vi "Idle_Password.vi"(2 "Called?":bool=TRUE) -> (0 "Correct?":bool, 1 "Access Level":i32)   [LabVIEW 2012]
uses:
  WVDIAL_GlobalVariables.vi
  <vilib>/Utility/miscctls.llb/LVPointTypeDef.ctl
  <vilib>/Utility/miscctls.llb/LVRectTypeDef.ctl
panel:
  in  "Cancel":bool
  in  "Password":string
  in  "Set Password":bool
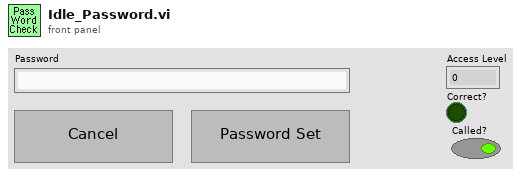
[diagram p1: front panel]
types:
  T1 = typedef "LVPointTypeDef.ctl" = cluster{"Horizontal":i16, "Vertical":i16}
  T2 = typedef "LVRectTypeDef.ctl" = cluster{"Left":i16, "Top":i16, "Right":i16, "Bottom":i16}
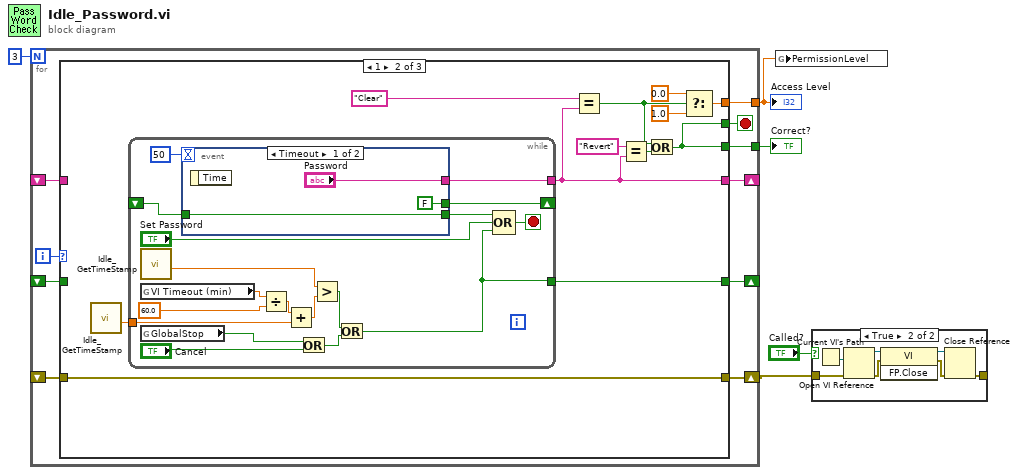
[diagram p0: block diagram]
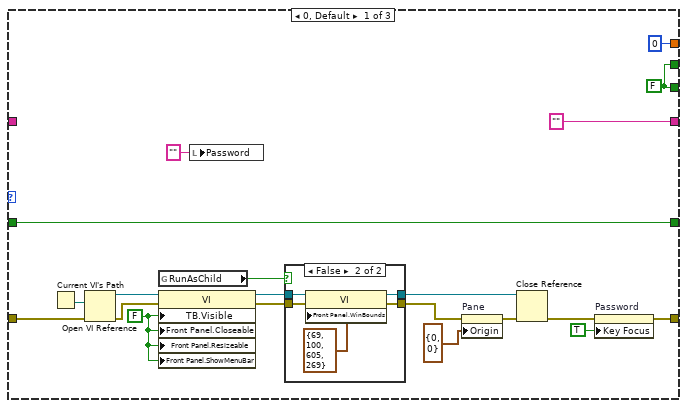
[diagram p3: hidden frame]
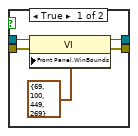
[diagram p4: hidden frame]
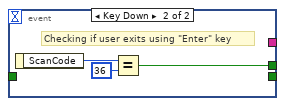
[diagram p5: hidden frame]
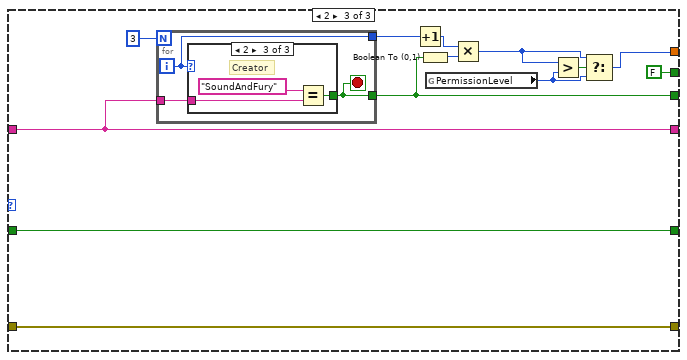
[diagram p6: hidden frame]
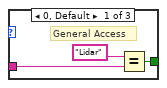
[diagram p7: hidden frame]
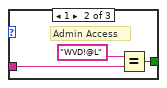
[diagram p8: hidden frame]
diagram:
  n1 = for {
    N: 3 -> [_]
    shift-right: [w14] -> _
    shift-left: _ -> [w11]
    shift-right: [w13] -> _
    shift-left: _ -> [w12]
    shift-right: [w9] -> w2
    shift-left: _ -> [w10]
    tunnel: [w8] -> w3
    tunnel: [w7] -> w4
    i -> [w15]
    stop <- w6 stop-if-true
    n2 = case shown="1" w15 {
      tunnel: ["" ("Comment") w53 w93] -> w14
      tunnel: [w32 w56 w94] -> w13
      tunnel: w12 -> [w32 _ w94]
      tunnel: w11 -> [_ _ w93]
      tunnel: w10 -> [w31 w46 w82]
      tunnel: [w17 w46 w82] -> w9
      tunnel: [w28 w47 w89] -> w7
      tunnel: [0 w51 w85] -> w8
      tunnel: [w28 w47 FALSE] -> w6
      frame 0, Default {
        w28 = FALSE
        w35 = FALSE ("Tool Bar:Visible")
        n3 = Current VI's Path() -> (path=w34:path)
        n4 = Open VI Reference(vi path=w34, error in (no error)=w31) -> (vi reference=w20:refnum<vi>, error out=w19:errorcluster)  [unwired: 4 in]
        n5 = global read "WVDIAL_GlobalVariables.vi" "RunAsChild"() -> (w21:bool)
        n6 = property class="VI"(reference=w20, error in=w19, "TB.Visible"=w35, "Front Panel.Closeable"=w35, "Front Panel.Resizeable"=w35, "Front Panel.ShowMenuBar"=w35) -> (reference out=w25:refnum<vi>, error out=w23:errorcluster)
        n7 = local write "Password"("" ("Password")) -> ()
        n8 = case shown="False" w21 {
          tunnel: w25 -> [w40 w45]
          tunnel: [w39 w44] -> w24
          tunnel: w23 -> [w38 w43]
          tunnel: [w37 w42] -> w22
          frame True {
            n9 = property class="VI"(reference=w40, error in=w38, "Front Panel.WinBounds"=T2 {"Left"=69, "Top"=100, "Right"=449, "Bottom"=269} ("Front Panel Window:Window Bounds 2")) -> (reference out=w39:refnum<vi>, error out=w37:errorcluster)
          }
          frame False {
            n10 = property class="VI"(reference=w45, error in=w43, "Front Panel.WinBounds"=T2 {"Left"=69, "Top"=100, "Right"=605, "Bottom"=269} ("Front Panel Window:Window Bounds 2")) -> (reference out=w44:refnum<vi>, error out=w42:errorcluster)
          }
        }
        n11 = property on="Pane" class="Pane"(error in=w22, "Origin"=T1 {"Horizontal"=0, "Vertical"=0}) -> (error out=w27:errorcluster)  [unwired: 1 in, 1 out]
        n12 = Close Reference(reference=w24, error in (no error)=w27) -> (error out=w18:errorcluster)
        n13 = property on="Password" class="Str"(error in=w18, "Key Focus"=TRUE) -> (error out=w17:errorcluster)  [unwired: 1 in, 1 out]
      }
      frame 1 {
        n14 = call "Idle_GetTimeStamp.vi"() -> ("Fractional Hours"=w57:dbl)  [unwired: 11 in]
        n15 = while {
          tunnel: w57 -> [w71]
          tunnel: [w63] -> w56
          shift-right: [w60] -> _
          shift-left: _ -> [w59]
          tunnel: [w61] -> w53
          stop <- w64 stop-if-true
          n16 = call "Idle_GetTimeStamp.vi"() -> ("Fractional Hours"=w75:dbl)  [unwired: 11 in]
          n17 = global read "WVDIAL_GlobalVariables.vi" "VI Timeout (min)"() -> (w67:dbl)
          n18 = global read "WVDIAL_GlobalVariables.vi" "GlobalStop"() -> (w66:bool)
          n19 = event shown="[0] Timeout" {
            selector: _ -> [_ _]
            dyn-events: _ -> [_ _]
            timeout: 50 -> [_ _]
            tunnel: ["Password" _] -> w61
            tunnel: [FALSE w79] -> w60
            tunnel: w59 -> [w77 _]
            tunnel: [w77 _] -> w58
            event Timeout {
              n20 = event-data() -> ()  [unwired: 1 in, 1 out]
            }
            event Key Down {
              # "Checking if user exits using \"Enter\" key"
              n21 = event-data() -> ("ScanCode"=w81:i16)  [unwired: 1 in]
              n22 = Equal?(x=w81, y=i16 36) -> (x = y?=w79:bool)
            }
          }
          n23 = Divide(x=w67, y=60.0) -> (x/y=w72:dbl)
          n24 = Add(x=w72, y=w71) -> (x+y=w74:dbl)
          n25 = Or(x=w66, y="Cancel") -> (x .or. y?=w68:bool)
          n26 = Greater?(x=w75, y=w74) -> (0:w70:bool)
          n27 = Or(x=w70, y=w68) -> (x .or. y?=w63:bool)
          n28 = Compound Arithmetic op=OR(w58, "Set Password", w63) -> (w64:bool)
        }
        n29 = Equal?(x="Clear" ("y"), y=w53) -> (x = y?=w48:bool)
        n30 = Equal?(x="Revert" ("y"), y=w53) -> (x = y?=w52:bool)
        n31 = Or(x=w48, y=w52) -> (x .or. y?=w47:bool)
        n32 = Select(t=0.0, s=w48, f=1.0) -> (s? t:f=w51:dbl)
      }
      frame 2 {
        n33 = for {
          N: 3 -> [_]
          tunnel: w93 -> [w97]
          tunnel: [w96] -> w89
          tunnel: [w95] -> w91
          i -> [w95]
          stop <- w96 stop-if-true
          n34 = case shown="2" w95 {
            tunnel: w97 -> [w98 w101 w104]
            tunnel: [w99 w102 w105] -> w96
            frame 0, Default {
              # "General Access"
              n35 = Equal?(x="Lidar", y=w98) -> (x = y?=w99:bool)
            }
            frame 1 {
              # "Admin Access"
              n36 = Equal?(x="WVD!@L", y=w101) -> (x = y?=w102:bool)
            }
            frame 2 {
              # "Creator"
              n37 = Equal?(x="SoundAndFury", y=w104) -> (x = y?=w105:bool)
            }
          }
        }
        n38 = Increment(x=w91) -> (x+1=w90:i32)
        n39 = Boolean To (0,1)(Boolean=w89) -> (0, 1=w88:i16)
        n40 = global read "WVDIAL_GlobalVariables.vi" "PermissionLevel"() -> (w83:i32)
        n41 = Multiply(x=w90, y=w88) -> (x*y=w86:i32)
        n42 = Greater?(x=w86, y=w83) -> (0:w87:bool)
        n43 = Select(t=w86, s=w87, f=w83) -> (s? t:f=w85:i32)
      }
    }
  }
  "Correct?" <- w4
  "Access Level" <- w3
  n44 = global write "WVDIAL_GlobalVariables.vi" "PermissionLevel"(w3) -> ()
  n45 = case shown="True" "Called?" {
    tunnel: w2 -> [w107 w109]
    tunnel: [w107 w108] -> _
    frame False {
    }
    frame True {
      n46 = Current VI's Path() -> (path=w114:path)
      n47 = Open VI Reference(vi path=w114, error in (no error)=w109) -> (vi reference=w113:refnum<vi>, error out=w112:errorcluster)  [unwired: 4 in]
      n48 = invoke on="Invoke Node" class="VI" method="FP.Close"(reference=w113, error in=w112) -> (reference out=w110:refnum<vi>, error out=w111:errorcluster)  [unwired: 1 in, 1 out]
      n49 = Close Reference(reference=w110, error in (no error)=w111) -> (error out=w108:errorcluster)
    }
  }
